vi "uso de subVI.vi"() -> ()   [LabVIEW 2020]
panel:
  out "Termometro":dbl(slide) scale=0.0..120.0
  out "C":bool
  out "F":bool
  in  "Seletor de unidade":bool
  in  "Sinal do sensor":dbl(knob) scale=0.0..5.0
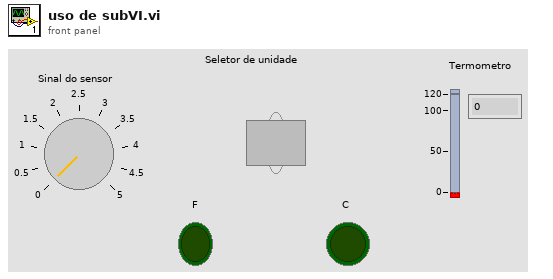
[diagram p1: front panel]
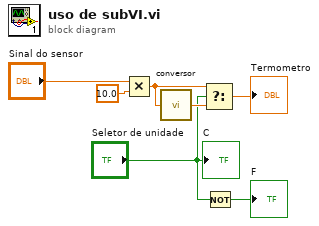
[diagram p0: block diagram]
diagram:
  n1 = Multiply(x="Sinal do sensor", y=10.0) -> (x*y=w5:dbl)
  n2 = call "conversor.vi"("Temperatura (C)"=w5) -> ("Temperatura (F)"=w4:dbl)
  n3 = Select(t=w5, s="Seletor de unidade", f=w4) -> (s? t:f=→"Termometro":dbl)
  n4 = Not(x="Seletor de unidade") -> (.not. x?=→"F":bool)
  "C" <- "Seletor de unidade"
